vi "simulated ixon.vi"(8 "error in (no error)":errorcluster) -> (0 "error out":errorcluster)   [LabVIEW 2018]
uses:
  Sim_Ixon_Ultra/Sim_Ixon_Ultra.lvclass
  C:/Users/Denis/Desktop/S4ACS/S4ACS/Sim_CCD/Sim_CCD.lvclass
  <vilib>/addons/_JKI Toolkits/Caraya/classes/Assert/Assert Equal Value_Variant.vi
  <vilib>/addons/_JKI Toolkits/Caraya/classes/Test/Test.lvclass
  <vilib>/addons/_JKI Toolkits/Caraya/classes/Assert/Assert.lvclass
  Sim_CCD/Sim_CCD.lvclass
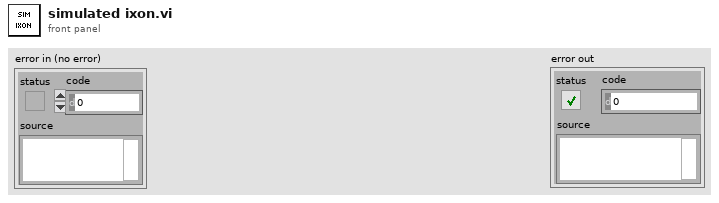
[diagram p1: front panel]
types:
  T1 = cluster{"EM_MODE":u16, "EM_GAIN":u16, "FRAME_TRANSFER":bool}
  T2 = cluster{"PREAMP":u16, "READOUT_RATE":u16, "VERTICAL_SHIFT_SPEED":u16, "READ_MODE":u16, "VERTICAL_CLOCK_VOLTAGE":u16, "ACQUISITION_MODE":u16, "AD_CHANNEL":u16, "SHUTTER_TTL":u16, "SHUTTER_OPENING_TIME":u16, "SHUTTER_CLOSING_TIME":u16, "SHUTTER_MODE":u16, "TRIGGER_MODE":u16, "VBIN":u16, "INITIAL_LINE":u16, "INITIAL_COLUMN":u16, "FINAL_LINE":u16, "FINAL_COLUMN":u16, "HBIN":u16}
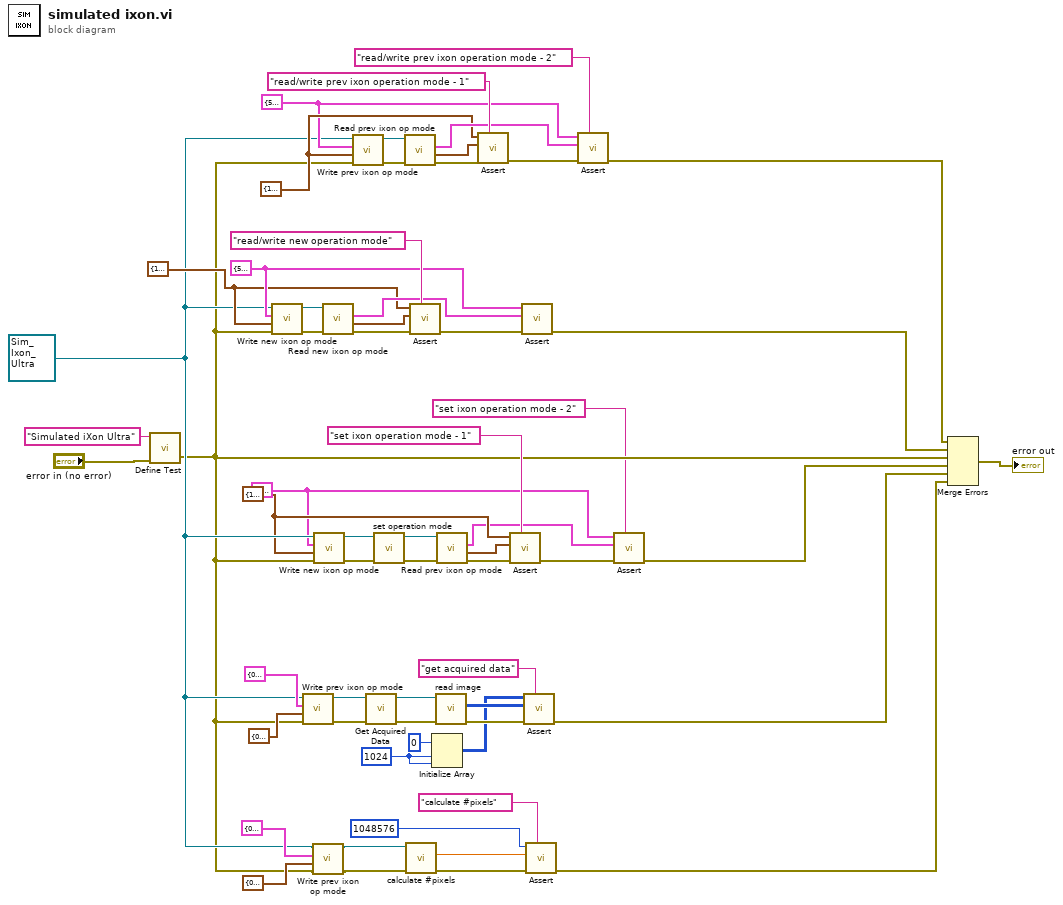
[diagram p0: block diagram]
diagram:
  w6 = T1 {"EM_MODE"=5, "EM_GAIN"=3, "FRAME_TRANSFER"=TRUE} ("prev ixon op mode")
  w8 = T2 {"PREAMP"=1, "READOUT_RATE"=2, "VERTICAL_SHIFT_SPEED"=3, "READ_MODE"=4, "VERTICAL_CLOCK_VOLTAGE"=5, "ACQUISITION_MODE"=6, "AD_CHANNEL"=7, "SHUTTER_TTL"=8, "SHUTTER_OPENING_TIME"=9, "SHUTTER_CLOSING_TIME"=11, "SHUTTER_MODE"=12, "TRIGGER_MODE"=13, "VBIN"=14, "INITIAL_LINE"=15, "INITIAL_COLUMN"=16, "FINAL_LINE"=17, "FINAL_COLUMN"=18, "HBIN"=19} ("prev operation mode")
  w20 = T1 {"EM_MODE"=5, "EM_GAIN"=3, "FRAME_TRANSFER"=TRUE} ("prev ixon op mode")
  w19 = T2 {"PREAMP"=1, "READOUT_RATE"=2, "VERTICAL_SHIFT_SPEED"=3, "READ_MODE"=4, "VERTICAL_CLOCK_VOLTAGE"=5, "ACQUISITION_MODE"=6, "AD_CHANNEL"=7, "SHUTTER_TTL"=8, "SHUTTER_OPENING_TIME"=9, "SHUTTER_CLOSING_TIME"=11, "SHUTTER_MODE"=12, "TRIGGER_MODE"=13, "VBIN"=14, "INITIAL_LINE"=15, "INITIAL_COLUMN"=16, "FINAL_LINE"=17, "FINAL_COLUMN"=18, "HBIN"=19} ("prev operation mode")
  w27 = T1 {"EM_MODE"=5, "EM_GAIN"=3, "FRAME_TRANSFER"=TRUE} ("prev ixon op mode")
  w28 = T2 {"PREAMP"=1, "READOUT_RATE"=2, "VERTICAL_SHIFT_SPEED"=3, "READ_MODE"=4, "VERTICAL_CLOCK_VOLTAGE"=5, "ACQUISITION_MODE"=6, "AD_CHANNEL"=7, "SHUTTER_TTL"=8, "SHUTTER_OPENING_TIME"=9, "SHUTTER_CLOSING_TIME"=11, "SHUTTER_MODE"=12, "TRIGGER_MODE"=13, "VBIN"=14, "INITIAL_LINE"=15, "INITIAL_COLUMN"=16, "FINAL_LINE"=17, "FINAL_COLUMN"=18, "HBIN"=19} ("prev operation mode")
  w13 = refnum<class "Sim_Ixon_Ultra.lvclass"> refnum ("Sim_Ixon_Ultra.lvclass")
  w51 = 1024 ("dimension size")
  n1 = call <vilib>:"Define Test.vi"("error in (no error)"="error in (no error)", "Label (VI Title)"="Simulated iXon Ultra") -> ("error out"=w12:errorcluster)  [unwired: 8 in, 1 out]
  n2 = call-dynamic "Write new ixon op mode.vi"("error in (no error)"=w12, "new operation mode"=w19, "new ixon op mode"=w20, "Sim_Ixon_Ultra in"=w13) -> ("error out"=w25:errorcluster, "Sim_Ixon_Ultra out"=w24:refnum<class "Sim_Ixon_Ultra.lvclass">)  [unwired: 6 in]
  n3 = call-dynamic "Write prev ixon op mode.vi"("error in (no error)"=w12, "prev operation mode"=T2 {"PREAMP"=0, "READOUT_RATE"=0, "VERTICAL_SHIFT_SPEED"=0, "READ_MODE"=0, "VERTICAL_CLOCK_VOLTAGE"=0, "ACQUISITION_MODE"=0, "AD_CHANNEL"=0, "SHUTTER_TTL"=0, "SHUTTER_OPENING_TIME"=0, "SHUTTER_CLOSING_TIME"=0, "SHUTTER_MODE"=0, "TRIGGER_MODE"=0, "VBIN"=1, "INITIAL_LINE"=1, "INITIAL_COLUMN"=1, "FINAL_LINE"=1024, "FINAL_COLUMN"=1024, "HBIN"=1}, "prev ixon op mode"=T1 {"EM_MODE"=0, "EM_GAIN"=2, "FRAME_TRANSFER"=FALSE}, "Sim_Ixon_Ultra in"=w13) -> ("error out"=w40:errorcluster, "Sim_Ixon_Ultra out"=w39:refnum<class "Sim_Ixon_Ultra.lvclass">)  [unwired: 6 in]
  n4 = call-dynamic "Write prev ixon op mode.vi"("error in (no error)"=w12, "prev operation mode"=T2 {"PREAMP"=0, "READOUT_RATE"=0, "VERTICAL_SHIFT_SPEED"=0, "READ_MODE"=0, "VERTICAL_CLOCK_VOLTAGE"=0, "ACQUISITION_MODE"=0, "AD_CHANNEL"=0, "SHUTTER_TTL"=0, "SHUTTER_OPENING_TIME"=0, "SHUTTER_CLOSING_TIME"=0, "SHUTTER_MODE"=0, "TRIGGER_MODE"=0, "VBIN"=1, "INITIAL_LINE"=1, "INITIAL_COLUMN"=1, "FINAL_LINE"=1024, "FINAL_COLUMN"=1024, "HBIN"=1}, "prev ixon op mode"=T1 {"EM_MODE"=0, "EM_GAIN"=2, "FRAME_TRANSFER"=FALSE}, "Sim_Ixon_Ultra in"=w13) -> ("error out"=w43:errorcluster, "Sim_Ixon_Ultra out"=w42:refnum<class "Sim_Ixon_Ultra.lvclass">)  [unwired: 6 in]
  n5 = call-dynamic "Write new ixon op mode.vi"("error in (no error)"=w12, "new operation mode"=w8, "new ixon op mode"=w6, "Sim_Ixon_Ultra in"=w13) -> ("error out"=w14:errorcluster, "Sim_Ixon_Ultra out"=w15:refnum<class "Sim_Ixon_Ultra.lvclass">)  [unwired: 6 in]
  n6 = call-dynamic "Read new ixon op mode.vi"("error in (no error)"=w25, "Sim_Ixon_Ultra in"=w24) -> ("error out"=w26:errorcluster, "new operation mode"=w23:T2, "new ixon op mode"=w21:T1)  [unwired: 6 in, 1 out]
  n7 = call-dynamic "Write prev ixon op mode.vi"("error in (no error)"=w12, "prev operation mode"=w28, "prev ixon op mode"=w27, "Sim_Ixon_Ultra in"=w13) -> ("error out"=w35:errorcluster, "Sim_Ixon_Ultra out"=w34:refnum<class "Sim_Ixon_Ultra.lvclass">)  [unwired: 6 in]
  n8 = call-dynamic "Get Acquired Data.vi"("error in (no error)"=w40, "CCDCamera in"=w39) -> ("error out"=w54:errorcluster, "CCDCamera out"=w55:refnum<class "Sim_Ixon_Ultra.lvclass">)  [unwired: 8 in]
  n9 = call-dynamic "set operation mode.vi"("error in (no error)"=w14, "CCDCamera in"=w15) -> ("error out"=w16:errorcluster, "CCDCamera out"=w17:refnum<class "Sim_Ixon_Ultra.lvclass">)  [unwired: 8 in]
  n10 = call-dynamic "Read prev ixon op mode.vi"("error in (no error)"=w35, "Sim_Ixon_Ultra in"=w34) -> ("error out"=w33:errorcluster, "prev operation mode"=w32:T2, "prev ixon op mode"=w30:T1)  [unwired: 6 in, 1 out]
  n11 = call "calculate #pixels.vi"("error in (no error)"=w43, "Simulated Camera in"=w42) -> ("error out"=w47:errorcluster, "#pixels"=w46:dbl)  [unwired: 7 in, 1 out]
  n12 = call-poly <vilib>:"Assert.vi"("Label"="read/write new operation mode", "error in (no error)"=w26, "Actual"=w23, "Expected"=w19) -> ("error out"=w22:errorcluster)  [unwired: 6 in, 1 out]
  n13 = Initialize Array(u16 0, w51, w51) -> (w49:u16[][])
  n14 = call "read image.vi"("error in (no error)"=w54, "CCDCamera in"=w55) -> ("error out"=w52:errorcluster, "Image Graph"=w50:u16[][])  [unwired: 7 in, 1 out]
  n15 = call-dynamic "Read prev ixon op mode.vi"("error in (no error)"=w16, "Sim_Ixon_Ultra in"=w17) -> ("error out"=w18:errorcluster, "prev operation mode"=w9:T2, "prev ixon op mode"=w7:T1)  [unwired: 6 in, 1 out]
  n16 = call-poly <vilib>:"Assert.vi"("Label"="read/write prev ixon operation mode - 1", "error in (no error)"=w33, "Actual"=w32, "Expected"=w28) -> ("error out"=w31:errorcluster)  [unwired: 6 in, 1 out]
  n17 = call-poly <vilib>:"Assert.vi"("Label"="set ixon operation mode - 1" ("Label (VI Title)"), "error in (no error)"=w18, "Actual"=w9, "Expected"=w8) -> ("error out"=w11:errorcluster)  [unwired: 6 in, 1 out]
  n18 = call-poly <vilib>:"Assert.vi"("error in (no error)"=w22, "Actual"=w21, "Expected"=w20) -> ("error out"=w2:errorcluster)  [unwired: 7 in, 1 out]
  n19 = call-poly <vilib>:"Assert.vi"("Label"="get acquired data" ("Label (VI Title)"), "error in (no error)"=w52, "Actual"=w50, "Expected"=w49) -> ("error out"=w4:errorcluster)  [unwired: 6 in, 1 out]
  n20 = call-poly <vilib>:"Assert.vi"("Label"="calculate #pixels" ("Label (VI Title)"), "error in (no error)"=w47, "Actual"=w46, "Expected"=u32 1048576 ("y")) -> ("error out"=w3:errorcluster)  [unwired: 6 in, 1 out]
  n21 = call-poly <vilib>:"Assert.vi"("Label"="read/write prev ixon operation mode - 2", "error in (no error)"=w31, "Actual"=w30, "Expected"=w27) -> ("error out"=w1:errorcluster)  [unwired: 6 in, 1 out]
  n22 = call-poly <vilib>:"Assert.vi"("Label"="set ixon operation mode - 2" ("Label (VI Title)"), "error in (no error)"=w11, "Actual"=w7, "Expected"=w6) -> ("error out"=w10:errorcluster)  [unwired: 6 in, 1 out]
  n23 = Merge Errors(w1, w2, w12, w10, w4, w3) -> (→"error out":errorcluster)
